vi "19.2.1-1D Barcode.vi"() -> ()   [LabVIEW 2017]
doc: "This example shows how to use the IMAQ Read Barcode VI to locate and read standard 1D barcodes."
uses:
  <vilib>/vision/Instrument.llb/Barcode Search Options.ctl
  <vilib>/vision/NI_Vision_Development_Module.lvlib
panel:
  out "Barcode ANSI/CEN/ISO Grading Report":T1(array[cluster])
  out "Barcode Read":cluster{"Data":string, "Barcode Type":string}[](array[cluster])
  out "Number of Barcodes Found":u32
  out "Image":T2(plugin-control)
  in  "Delay (s.)":dbl(slide)=0.4897959183673469 scale=0.0..2.0
  in  "Stop":bool
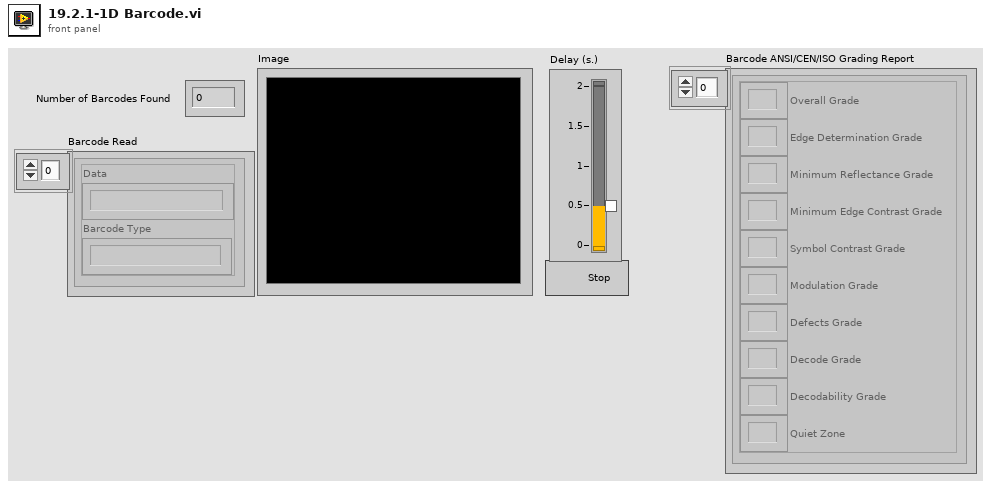
[diagram p1: front panel]
types:
  T1 = cluster{"Overall Grade":string, "Edge Determination Grade":string, "Minimum Reflectance Grade":string, "Minimum Edge Contrast Grade":string, "Symbol Contrast Grade":string, "Modulation Grade":string, "Defects Grade":string, "Decode Grade":string, "Decodability Grade":string, "Quiet Zone":string}[]
  T2 = typedef "IMAQ Image.ctl" = refnum<image>
  T3 = cluster{"Calculate Grading Report":bool, "Scan Width ":i32}
  T4 = typedef "Barcode Search Options.ctl" = cluster{"Min Bar Width":u32, "Min Edge Strength":u32, "Min Bars":u32, "Skip Location Search?":bool}
  T5 = cluster{"Data":string, "Special Char 1":string, "Special Char 2":string, "Checksum(s)":string, "Barcode Type":u32, "Confidence Level":sgl, "Bounding Box":cluster{"x":sgl, "y":sgl}[]}[]
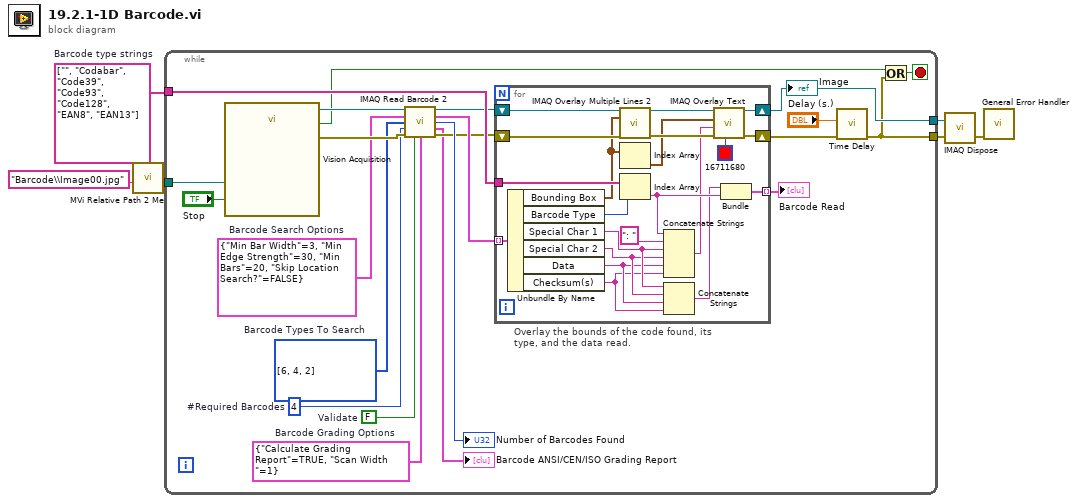
[diagram p0: block diagram]
diagram:
  w5 = string[] ["", "Codabar", "Code39", "Code93", "Code128", "EAN8", "EAN13"]  # Barcode type strings
  n1 = call "MVi Relative Path 2 Me.vi"("Relative Path"="Barcode\\Image00.jpg") -> ("Appended Dir"=w1:path)  [unwired: 5 in, 1 out]
  n2 = while {
    tunnel: [w14] -> w6
    tunnel: [w7] -> w4
    tunnel: w1 -> [w26]
    tunnel: w5 -> [w22]
    stop <- w28 stop-if-true
    w11 = T3 {"Calculate Grading Report"=TRUE, "Scan Width "=1}  # Barcode Grading Options
    w12 = T4 {"Min Bar Width"=3, "Min Edge Strength"=30, "Min Bars"=20, "Skip Location Search?"=FALSE}  # Barcode Search Options
    w24 = u32 4  # #Required Barcodes
    w18 = u32[] [6, 4, 2] items=["Reserved", "Codabar", "Code 39", "Code 93", "Code 128", "EAN 8", "EAN 13", "Interleaved 2 of 5", "MSI", "UPCA", "Pharmacode", "RSS Limited"]  # Barcode Types To Search
    w13 = FALSE  # Validate
    # "Overlay the bounds of the code found, its type, and the data read."
    n3 = call "Vision Acquisition"("Image Path"=w26, "Stop (F)"="Stop") -> ("Image Out"=w20:T2, "Stopped"=w8:bool, "error out"=w25:errorcluster)  [unwired: 23 in]
    n4 = call "IMAQ Read Barcode 2"("Image"=w20, "Barcode Search Options"=w12, "Barcode Types To Search"=w18, "Num of Required Barcodes"=w24, "error in (no error)"=w25, "Validate"=w13, "Barcode Grading Options"=w11) -> ("Image (duplicate)"=w21:T2, "Barcodes"=w23:T5, "Num of Barcodes"=→"Number of Barcodes Found":u32, "Barcode ANSI/CEN/ISO Grading Report"=→"Barcode ANSI/CEN/ISO Grading Report":T1, "error out"=w17:errorcluster)  [unwired: 4 in]
    n5 = for {
      tunnel: w23 -> [w49] mode=indexing
      tunnel: w22 -> [w48]
      shift-right: [w44] -> w14
      shift-left: w21 -> [w40]
      shift-right: [w41] -> w16
      shift-left: w17 -> [w43]
      tunnel: [w36] -> w10 mode=indexing
      n6 = Unbundle By Name(w49) -> ("Bounding Box"=w39:cluster{"x":sgl, "y":sgl}[], "Barcode Type"=w37:u32, "Special Char 1"=w33:string, "Special Char 2"=w32:string, "Data"=w31:string, "Checksum(s)"=w30:string)
      n7 = call "IMAQ Overlay Multiple Lines 2"("Image"=w40, "Line End Points"=w39, "error in (no error)"=w43) -> ("Image Out"=w46:T2, "error out"=w42:errorcluster)  [unwired: 11 in]
      n8 = Index Array(array=w39) -> (element=w38:cluster{"x":sgl, "y":sgl})  [unwired: 1 in]
      n9 = Index Array(array=w48, index=w37) -> (element=w35:string)
      n10 = Concatenate Strings(w35, ": " ("string"), w33, w32, w31, w30) -> (w34:string)
      n11 = Concatenate Strings(w33, w32, w31, w30) -> (w29:string)
      n12 = call "IMAQ Overlay Text"("Text Color (black)"=u32 16711680, "error in (no error)"=w42, "String"=w34, "Origin"=w38, "Image"=w46) -> ("error out"=w41:errorcluster, "Image Out"=w44:T2)  [unwired: 5 in]
      n13 = Bundle(w29, w35) -> (w36:cluster{string, string})  [unwired: 1 in]
    }
    "Image" <- w14
    "Barcode Read" <- w10
    n14 = call "Time Delay"("error in (no error)"=w16, "Delay Time (s)"="Delay (s.)") -> ("error out"=w7:errorcluster)  [unwired: 9 in]
    n15 = Or(x=w8, y=w7) -> (x .or. y?=w28:bool)
  }
  n16 = call "IMAQ Dispose"("Image"=w6, "error in (no error)"=w4) -> ("error out"=w3:errorcluster)  [unwired: 1 in, 3 out]
  n17 = call <vilib>:"General Error Handler.vi"("error in (no error)"=w3) -> ()  [unwired: 10 in, 5 out]
